vi "ExTestPutU16.vi"() -> ()   [LabVIEW 2010]
panel:
  out "Image Display 2":u16[][](graph)
  out "error out":errorcluster
  in  "error in (no error)":errorcluster
  out "Image Display":i32[][](graph)
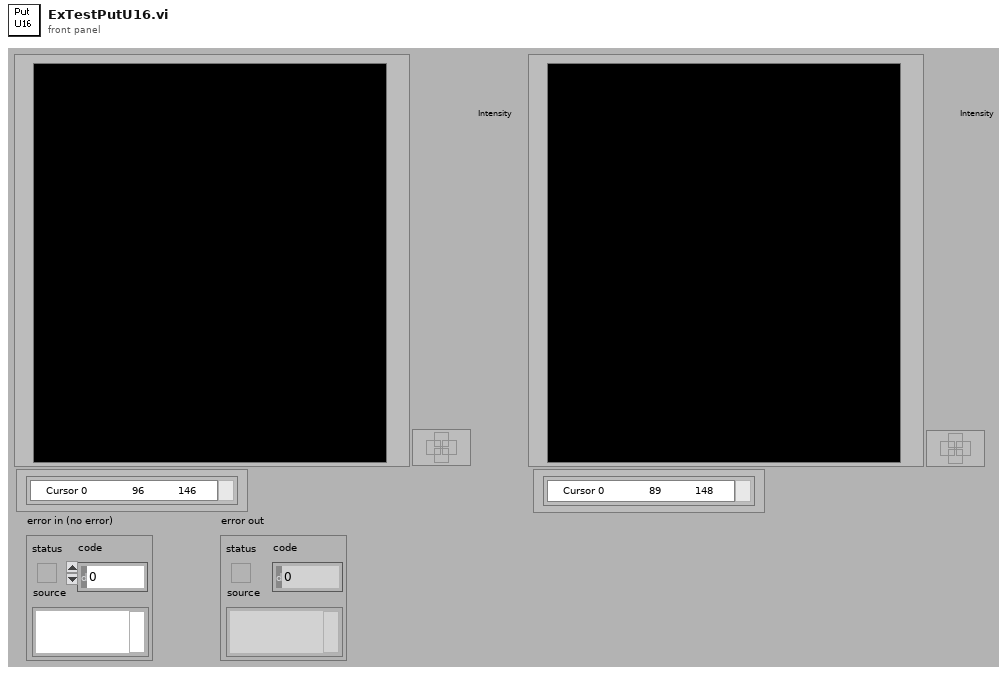
[diagram p1: front panel]
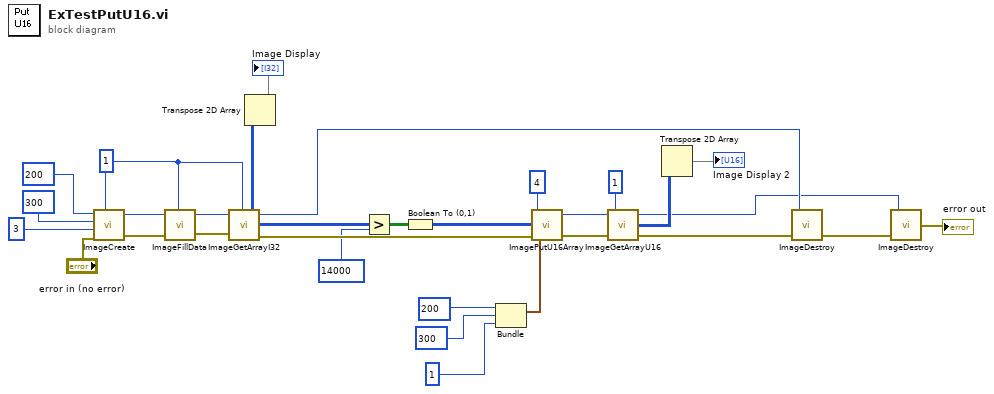
[diagram p0: block diagram]
diagram:
  w21 = 1
  n1 = call <userlib>:"ImageCreate.vi"("X dimension"=200, "Y dimension"=300, "Data Type"=3, "error in"="error in (no error)", "Number Of Frames"=w21) -> ("Image Handle"=w25:u32, "error out"=w26:errorcluster)
  n2 = call <userlib>:"ImageFillData.vi"("error in"=w26, "Type of Test"=w21, "Image Handle"=w25) -> ("error out"=w24:errorcluster, "Image Handle"=w23:u32)
  n3 = call <userlib>:"ImageGetArrayI32.vi"("error in"=w24, "Z position"=w21, "Image Handle"=w23) -> ("error out"=w19:errorcluster, "Array int 32"=w4:i32[][], "Image Handle"=w13:u32)
  n4 = Transpose 2D Array(2D array=w4) -> (transposed array=→"Image Display":i32[][])
  n5 = Greater?(x=w4, y=14000) -> (0:w2:bool[][])
  n6 = Boolean To (0,1)(Boolean=w2) -> (0, 1=w1:i16[][])
  n7 = Bundle(200, 300, 1) -> (w8:cluster{i32, i32, i32})  [unwired: 1 in]
  n8 = call <userlib>:"ImagePutU16Array.vi"("error in (no error)"=w19, "Image dimensions"=w8, "Image Data"=w1, "Data Type to store as"=4) -> ("error out"=w18:errorcluster, "Image Handle"=w17:u32)
  n9 = call <userlib>:"ImageGetArrayU16.vi"("error in"=w18, "Z position"=1, "Image Handle"=w17) -> ("error out"=w12:errorcluster, "Array uint 16"=w15:u16[][], "Image Handle"=w10:u32)
  n10 = Transpose 2D Array(2D array=w15) -> (transposed array=→"Image Display 2":u16[][])
  n11 = call <userlib>:"ImageDestroy.vi"("error in"=w12, "Data handle"=w13) -> ("error out"=w11:errorcluster)
  n12 = call <userlib>:"ImageDestroy.vi"("error in"=w11, "Data handle"=w10) -> ("error out"=→"error out":errorcluster)
